vi "WPI_CameraBackground Loop_EDIT.vi"(0 "Front CameraDevRef":T1, 1 "Rear CameraDevRef":T1) -> ()   [LabVIEW 2015]
doc: "This VI acquires the image buffer from the camera MJPG stream at the configured fps rate. It notifies any waiting VIs and allows them to pick up the latest image. This allows the camera and robot vision loop to run at different rates. The 1011, camera is far more efficient using MJPGs, and generally, this is probably the better choice for the camera loop.\n \nThis software is licensed. Open the labview\\readme\\WPI Robotics Library Open Source License.txt file for more information."
uses:
  <vilib>/Rock Robotics/WPI/Camera/WPI_CameraDevRef.ctl
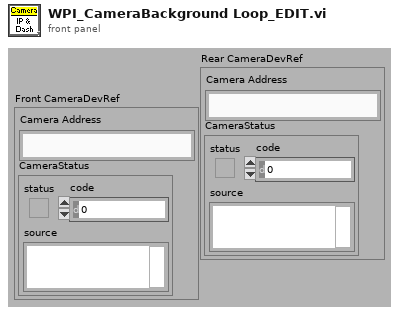
[diagram p1: front panel]
types:
  T1 = typedef "WPI_CameraDevRef.ctl" = cluster{"Camera Address":string, "CameraStatus":errorcluster}
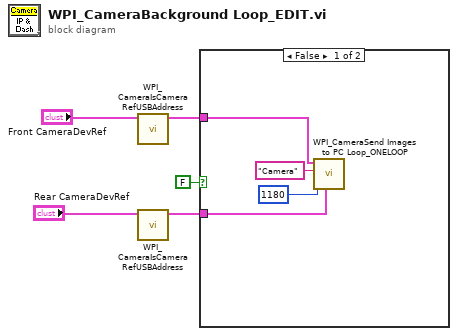
[diagram p0: block diagram]
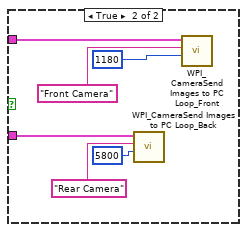
[diagram p2: hidden frame]
diagram:
  n1 = call <vilib>:"WPI_CameraIsCameraRefUSBAddress.vi"("CameraDevRef"="Front CameraDevRef") -> ("CameraDevRef out"=w2:T1)  [unwired: 7 in, 3 out]
  n2 = call <vilib>:"WPI_CameraIsCameraRefUSBAddress.vi"("CameraDevRef"="Rear CameraDevRef") -> ("CameraDevRef out"=w3:T1)  [unwired: 7 in, 3 out]
  n3 = case shown="False" FALSE {
    tunnel: w3 -> [w6 w15]
    tunnel: w2 -> [w9 w11]
    frame False {
      n4 = call "WPI_CameraSend Images to PC Loop_ONELOOP.vi"("CameraDevRef Back"=w6, "port"=u16 1180, "Image Name"="Camera", "CameraDevRef Front"=w9) -> ()  [unwired: 8 in]
    }
    frame True {
      n5 = call "WPI_CameraSend Images to PC Loop_Back.vi"("port"=u16 5800, "Image Name"="Rear Camera", "CameraDevRef"=w15) -> ()  [unwired: 9 in]
      n6 = call "WPI_CameraSend Images to PC Loop_Front.vi"("port"=u16 1180, "Image Name"="Front Camera", "CameraDevRef"=w11) -> ()  [unwired: 9 in]
    }
  }
